vi "RetoFor.vi"() -> ()   [LabVIEW 2022 SP3]
panel:
  out "Iteraciones":i32
  in  "Número a contar":i32
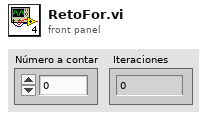
[diagram p1: front panel]
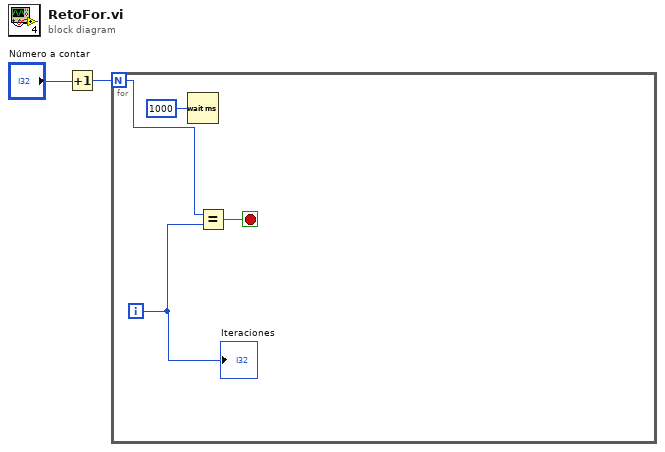
[diagram p0: block diagram]
diagram:
  n1 = Increment(x="Número a contar") -> (x+1=w2:i32)
  n2 = for {
    N: w2 -> [w6]
    i -> [w3]
    stop <- w5 stop-if-true
    n3 = Wait (ms)(milliseconds to wait=u32 1000) -> ()  [unwired: 1 out]
    n4 = Equal?(x=w6, y=w3) -> (x = y?=w5:bool)
    "Iteraciones" <- w3
  }
